vi "Untitled 1.vi"   [LabVIEW 2016]
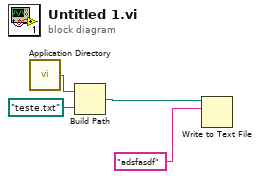
[diagram p0: block diagram]
diagram:
  n1 = call <vilib>:"Application Directory.vi"() -> ("Application Directory"=w4:path)
  n2 = Build Path(base path=w4, name or relative path=path "teste.txt" ("default name")) -> (appended path=w2:path)
  n3 = Write to Text File(file (use dialog)=w2, text="adsfasdf") -> ()  [unwired: 2 in, 3 out]
